vi "S4GUI_002.vi"(7 "Tab ObsEng":enum32{"Obs", "CCD modes", "Eng"}(tab)) -> ()   [LabVIEW 2018] (continued)
            n1697 = call "Write AcquisitionB.vi"("error in (no error)"=w3189, "Acquisition.lvclass"=w3190, "S4ACS_GUI in"=w3177) -> ("error out"=w3136:errorcluster, "S4ACS_GUI out"=w3135:refnum<class "S4GUI.lvclass">)  [unwired: 7 in]
            n1698 = call-dynamic "Read AcquisitionC.vi"("error in (no error)"=w3136, "S4ACS_GUI in"=w3135) -> ("error out"=w3173:errorcluster, "Acquisition.lvclass"=w3175:refnum<class "Acquisition.lvclass">, "S4ACS_GUI out"=w3176:refnum<class "S4GUI.lvclass">)  [unwired: 7 in]
            n1699 = call-dynamic "Read Channel.vi"("error in (no error)"=w3173, "Acquisition in"=w3175) -> ("error out"=w3160:errorcluster, "Channel.lvclass"=w3162:refnum<class "Channel.lvclass">, "Acquisition out"=w3174:refnum<class "Acquisition.lvclass">)  [unwired: 7 in]
            n1700 = call "Write section_name.vi"("error in (no error)"=w3160, "section_name"="CCD_ACS3", "Channel in"=w3162) -> ("error out"=w3159:errorcluster, "Channel out"=w3161:refnum<class "Channel.lvclass">)  [unwired: 7 in]
            n1701 = call-dynamic "load config.vi"("error in (no error)"=w3159, "cfg file name"=w3127, "Channel in"=w3161) -> ("error out"=w3117:errorcluster, "Channel out"=w3115:refnum<class "Channel.lvclass">)  [unwired: 7 in]
            n1702 = call-dynamic "save config.vi"("error in (no error)"=w3117, "file config"="lastsaved.cfg", "Channel in"=w3115) -> ("error out"=w3116:errorcluster, "Channel out"=w3114:refnum<class "Channel.lvclass">)  [unwired: 7 in]
            n1703 = call-dynamic "Read State Machine.vi"("error in (no error)"=w3116, "Device in"=w3114) -> ("error out"=w3169:errorcluster, "State Machine.lvclass"=w3171:refnum<class "State Machine.lvclass">, "Device out"=w3172:refnum<class "Channel.lvclass">)  [unwired: 7 in]
            n1704 = call-dynamic "Write State.vi"("error in (no error)"=w3169, "State"=60, "State Machine in"=w3171) -> ("error out"=w3168:errorcluster, "State Machine out"=w3170:refnum<class "State Machine.lvclass">)  [unwired: 7 in]
            n1705 = call-dynamic "Write State Machine.vi"("error in (no error)"=w3168, "State Machine.lvclass"=w3170, "Device in"=w3172) -> ("error out"=w3165:errorcluster, "Device out"=w3166:refnum<class "Channel.lvclass">)  [unwired: 7 in]
            n1706 = call-dynamic "Write Channel.vi"("error in (no error)"=w3165, "Channel.lvclass"=w3166, "Acquisition in"=w3174) -> ("error out"=w3164:errorcluster, "Acquisition out"=w3163:refnum<class "Acquisition.lvclass">)  [unwired: 7 in]
            n1707 = call-dynamic "Write AcquisitionC.vi"("error in (no error)"=w3164, "Acquisition.lvclass"=w3163, "S4ACS_GUI in"=w3176) -> ("error out"=w3134:errorcluster, "S4ACS_GUI out"=w3133:refnum<class "S4GUI.lvclass">)  [unwired: 7 in]
            n1708 = call-dynamic "Read AcquisitionD.vi"("error in (no error)"=w3134, "S4ACS_GUI in"=w3133) -> ("error out"=w3142:errorcluster, "Acquisition.lvclass"=w3140:refnum<class "Acquisition.lvclass">, "S4ACS_GUI out"=w3139:refnum<class "S4GUI.lvclass">)  [unwired: 7 in]
            n1709 = call-dynamic "Read Channel.vi"("error in (no error)"=w3142, "Acquisition in"=w3140) -> ("error out"=w3155:errorcluster, "Channel.lvclass"=w3153:refnum<class "Channel.lvclass">, "Acquisition out"=w3141:refnum<class "Acquisition.lvclass">)  [unwired: 7 in]
            n1710 = call "Write section_name.vi"("error in (no error)"=w3155, "section_name"="CCD_ACS4", "Channel in"=w3153) -> ("error out"=w3156:errorcluster, "Channel out"=w3154:refnum<class "Channel.lvclass">)  [unwired: 7 in]
            n1711 = call-dynamic "load config.vi"("error in (no error)"=w3156, "cfg file name"=w3127, "Channel in"=w3154) -> ("error out"=w3113:errorcluster, "Channel out"=w3111:refnum<class "Channel.lvclass">)  [unwired: 7 in]
            n1712 = call-dynamic "save config.vi"("error in (no error)"=w3113, "file config"="lastsaved.cfg", "Channel in"=w3111) -> ("error out"=w3112:errorcluster, "Channel out"=w3110:refnum<class "Channel.lvclass">)  [unwired: 7 in]
            n1713 = call-dynamic "Read State Machine.vi"("error in (no error)"=w3112, "Device in"=w3110) -> ("error out"=w3146:errorcluster, "State Machine.lvclass"=w3144:refnum<class "State Machine.lvclass">, "Device out"=w3143:refnum<class "Channel.lvclass">)  [unwired: 7 in]
            n1714 = call-dynamic "Write State.vi"("error in (no error)"=w3146, "State"=60, "State Machine in"=w3144) -> ("error out"=w3147:errorcluster, "State Machine out"=w3145:refnum<class "State Machine.lvclass">)  [unwired: 7 in]
            n1715 = call-dynamic "Write State Machine.vi"("error in (no error)"=w3147, "State Machine.lvclass"=w3145, "Device in"=w3143) -> ("error out"=w3150:errorcluster, "Device out"=w3149:refnum<class "Channel.lvclass">)  [unwired: 7 in]
            n1716 = call-dynamic "Write Channel.vi"("error in (no error)"=w3150, "Channel.lvclass"=w3149, "Acquisition in"=w3141) -> ("error out"=w3151:errorcluster, "Acquisition out"=w3152:refnum<class "Acquisition.lvclass">)  [unwired: 7 in]
            n1717 = call-dynamic "Write AcquisitionD.vi"("error in (no error)"=w3151, "Acquisition.lvclass"=w3152, "S4ACS_GUI in"=w3139) -> ("error out"=w3130:errorcluster, "S4ACS_GUI out"=w3132:refnum<class "S4GUI.lvclass">)  [unwired: 7 in]
            n1718 = Unbundle By Name(w3083) -> ("INITIAL_LINE"=w3104:u16, "INITIAL_COLUMN"=w3103:u16, "FINAL_LINE"=w3102:u16, "FINAL_COLUMN"=w3101:u16, "VBIN"=w3100:u16, "HBIN"=w3099:u16, "PREAMP"=w3098:u8, "EM_GAIN"=w3097:u16, "READOUT_RATE"=w3096:u8, "SHUTTER_OPENING_TIME"=w3095:u16, "SHUTTER_CLOSING_TIME"=w3094:u16, "VERTICAL_SHIFT_SPEED"=w3084:u8, "READ_MODE"=w3093:u8, "VERTICAL_CLOCK_VOLTAGE"=w3092:u8, "AD_CHANNEL"=w3091:u32, "SHUTTER_MODE"=w3090:u8, "SHUTTER_TTL"=w3089:u8, "TRIGGER_MODE"=w3088:u8, "FRAME_TRANSFER"=w3087:bool, "ACQUISITION_MODE"=w3086:u8, "EM_MODE"=w3085:u8)
            n1719 = call "Write cfg file.vi"("error in (no error)"=w3130, "cfg file"=w3127, "S4ACS_GUI in"=w3132) -> ("error out"=w3129:errorcluster, "S4ACS_GUI out"=w3131:refnum<class "S4GUI.lvclass">)  [unwired: 7 in]
            n1720 = local read "Input Cluster"() -> (w3106:T8)
            n1721 = Bundle By Name(cluster=w3106, "Parameters.Image \nInitial Line"=w3104, "Parameters.Image\nInitial Column"=w3103, "Parameters.Image\nFinal Line"=w3102, "Parameters.Image\nFInal Column"=w3101, "Parameters.Vertical\nBinning"=w3100, "Parameters.Horizontal\nBinning"=w3099, "Parameters.Pre-amplification\nGain"=w3098, "Parameters.CCD\nEM Gain"=w3097, "Parameters.Readout\nRate"=w3096, "Parameters.Shutter\nOpenning Time"=w3095, "Parameters.Shutter\nClosing Time"=w3094, "Parameters.Vertical\nShift Speed"=w3084, "Parameters.Read\nMode"=w3093, "Parameters.Vertical\nClock Voltage"=w3092, "Parameters.A/D \nChannel"=w3091, "Parameters.Shutter\nMode"=w3090, "Parameters.Shutter\nTTL"=w3089, "Parameters.Trigger\nMode"=w3088, "Parameters.Frame\nTransfer"=w3087, "Parameters.Acquisition\nMode"=w3086, "Parameters.CCD \nEM Mode"=w3085) -> (w3105:T8)
            n1722 = local write "Input Cluster"(w3105) -> ()
          }
          frame True {
          }
        }
      }
      event "Save As Button": Value Change {
        n1723 = event-data() -> ()  [unwired: 1 in, 6 out]
        n1724 = disable-structure shown="Enabled" {
          disable-tunnel: [w3231 w3243] -> w3220
          disable-tunnel: w3219 -> [w3230 _]
          disable-tunnel: [w3224 w3241] -> w3218
          frame Disabled {
            n1725 = String To Path(string="C:\\Users\\observer\\sparc4\\s4gui\\Config" ("default name")) -> (path=w3226:path)
            n1726 = call "File Dialog2"("start path"=w3226, "prompt"="Select file...", "button label"="Save", "default name"="lastsaved.cfg", "error in"=w3230, "pattern (all files)"="*.cfg") -> ("selected path"=w3225:path, "cancelled"=w3231:bool, "error out"=→"error out 3":errorcluster)  [unwired: 6 in, 1 out]
            n1727 = Strip Path(path=w3225) -> (name=w3224:string)  [unwired: 1 out]
          }
          frame Enabled {
            w3245 = ".cfg" ("regular expression")
            n1728 = Match Pattern(string="savefile", regular expression=w3245) -> (before substring=w3240:string, match substring=w3244:string)  [unwired: 1 in, 2 out]
            n1729 = String Length(string=w3240) -> (length=w3239:i32)
            n1730 = Equal?(x=w3244, y=w3245) -> (x = y?=w3235:bool)
            n1731 = Less?(x=w3239, y=20) -> (x < y?=w3236:bool)
            n1732 = And(x=w3236, y=w3235) -> (x .and. y?=w3237:bool)
            n1733 = case shown="False" w3237 {
              tunnel: w3240 -> [_ w3258]
              tunnel: w3244 -> [_ w3257]
              tunnel: [TRUE ("cancelled") FALSE ("cancelled")] -> w3243
              tunnel: [w3248 w3256] -> w3241
              tunnel: [w3248 w3256] -> w3242
              frame False {
                w3248 = "lastsaved.cfg" ("savefile")
                n1734 = One Button Dialog(message="Invalid file name!\nFile name length must be less than 20 characters\nand must contain .cfg ending." ("savefile")) -> ()  [unwired: 1 in, 1 out]
              }
              frame True {
                n1735 = call <vilib>:"Trim Whitespace.vi"("string"=w3258) -> ("trimmed string"=w3255:string)  [unwired: 1 in]
                n1736 = call <vilib>:"Space Constant.vi"() -> ("String"=w3253:string)
                n1737 = To Lower Case(string=w3255) -> (all lower case string=w3251:string)
                n1738 = Search and Replace String(replace all?=TRUE ("replace all? (F)"), input string=w3251, search string=w3253, replace string="" ("replace string (\"\")")) -> (result string=w3250:string)  [unwired: 4 in, 3 out]
                n1739 = Concatenate Strings(w3250, w3257) -> (w3256:string)
              }
            }
            n1740 = local write "savefile"(w3242) -> ()
          }
        }
        n1741 = case shown="False" w3220 {
          tunnel: w3223 -> [w3324 w3326]
          tunnel: [w3272 w3326] -> w3222
          tunnel: [w3270 w3325] -> w3221
          tunnel: w3219 -> [w3269 w3325]
          tunnel: w3218 -> [w3268 _]
          frame False {
            n1742 = call-dynamic "Read AcquisitionA.vi"("error in (no error)"=w3269, "S4ACS_GUI in"=w3324) -> ("error out"=w3320:errorcluster, "Acquisition.lvclass"=w3322:refnum<class "Acquisition.lvclass">, "S4ACS_GUI out"=w3323:refnum<class "S4GUI.lvclass">)  [unwired: 7 in]
            n1743 = call-dynamic "Read Channel.vi"("error in (no error)"=w3320, "Acquisition in"=w3322) -> ("error out"=w3315:errorcluster, "Channel.lvclass"=w3317:refnum<class "Channel.lvclass">, "Acquisition out"=w3321:refnum<class "Acquisition.lvclass">)  [unwired: 7 in]
            n1744 = call "Write section_name.vi"("error in (no error)"=w3315, "section_name"="CCD_ACS1", "Channel in"=w3317) -> ("error out"=w3314:errorcluster, "Channel out"=w3316:refnum<class "Channel.lvclass">)  [unwired: 7 in]
            n1745 = call-dynamic "save config.vi"("error in (no error)"=w3314, "file config"=w3268, "Channel in"=w3316) -> ("error out"=w3266:errorcluster, "Channel out"=w3267:refnum<class "Channel.lvclass">)  [unwired: 7 in]
            n1746 = call-dynamic "Write Channel.vi"("error in (no error)"=w3266, "Channel.lvclass"=w3267, "Acquisition in"=w3321) -> ("error out"=w3319:errorcluster, "Acquisition out"=w3318:refnum<class "Acquisition.lvclass">)  [unwired: 7 in]
            n1747 = call-dynamic "Write AcquisitionA.vi"("error in (no error)"=w3319, "Acquisition.lvclass"=w3318, "S4ACS_GUI in"=w3323) -> ("error out"=w3279:errorcluster, "S4ACS_GUI out"=w3278:refnum<class "S4GUI.lvclass">)  [unwired: 7 in]
            n1748 = call "Read AcquisitionB.vi"("error in (no error)"=w3279, "S4ACS_GUI in"=w3278) -> ("error out"=w3305:errorcluster, "Acquisition.lvclass"=w3303:refnum<class "Acquisition.lvclass">, "S4ACS_GUI out"=w3302:refnum<class "S4GUI.lvclass">)  [unwired: 7 in]
            n1749 = call-dynamic "Read Channel.vi"("error in (no error)"=w3305, "Acquisition in"=w3303) -> ("error out"=w3310:errorcluster, "Channel.lvclass"=w3308:refnum<class "Channel.lvclass">, "Acquisition out"=w3304:refnum<class "Acquisition.lvclass">)  [unwired: 7 in]
            n1750 = call "Write section_name.vi"("error in (no error)"=w3310, "section_name"="CCD_ACS2", "Channel in"=w3308) -> ("error out"=w3311:errorcluster, "Channel out"=w3309:refnum<class "Channel.lvclass">)  [unwired: 7 in]
            n1751 = call-dynamic "save config.vi"("error in (no error)"=w3311, "file config"=w3268, "Channel in"=w3309) -> ("error out"=w3260:errorcluster, "Channel out"=w3261:refnum<class "Channel.lvclass">)  [unwired: 7 in]
            n1752 = call-dynamic "Write Channel.vi"("error in (no error)"=w3260, "Channel.lvclass"=w3261, "Acquisition in"=w3304) -> ("error out"=w3306:errorcluster, "Acquisition out"=w3307:refnum<class "Acquisition.lvclass">)  [unwired: 7 in]
            n1753 = call "Write AcquisitionB.vi"("error in (no error)"=w3306, "Acquisition.lvclass"=w3307, "S4ACS_GUI in"=w3302) -> ("error out"=w3277:errorcluster, "S4ACS_GUI out"=w3276:refnum<class "S4GUI.lvclass">)  [unwired: 7 in]
            n1754 = call-dynamic "Read AcquisitionC.vi"("error in (no error)"=w3277, "S4ACS_GUI in"=w3276) -> ("error out"=w3298:errorcluster, "Acquisition.lvclass"=w3300:refnum<class "Acquisition.lvclass">, "S4ACS_GUI out"=w3301:refnum<class "S4GUI.lvclass">)  [unwired: 7 in]
            n1755 = call-dynamic "Read Channel.vi"("error in (no error)"=w3298, "Acquisition in"=w3300) -> ("error out"=w3293:errorcluster, "Channel.lvclass"=w3295:refnum<class "Channel.lvclass">, "Acquisition out"=w3299:refnum<class "Acquisition.lvclass">)  [unwired: 7 in]
            n1756 = call "Write section_name.vi"("error in (no error)"=w3293, "section_name"="CCD_ACS3", "Channel in"=w3295) -> ("error out"=w3292:errorcluster, "Channel out"=w3294:refnum<class "Channel.lvclass">)  [unwired: 7 in]
            n1757 = call-dynamic "save config.vi"("error in (no error)"=w3292, "file config"=w3268, "Channel in"=w3294) -> ("error out"=w3262:errorcluster, "Channel out"=w3263:refnum<class "Channel.lvclass">)  [unwired: 7 in]
            n1758 = call-dynamic "Write Channel.vi"("error in (no error)"=w3262, "Channel.lvclass"=w3263, "Acquisition in"=w3299) -> ("error out"=w3297:errorcluster, "Acquisition out"=w3296:refnum<class "Acquisition.lvclass">)  [unwired: 7 in]
            n1759 = call-dynamic "Write AcquisitionC.vi"("error in (no error)"=w3297, "Acquisition.lvclass"=w3296, "S4ACS_GUI in"=w3301) -> ("error out"=w3275:errorcluster, "S4ACS_GUI out"=w3274:refnum<class "S4GUI.lvclass">)  [unwired: 7 in]
            n1760 = call-dynamic "Read AcquisitionD.vi"("error in (no error)"=w3275, "S4ACS_GUI in"=w3274) -> ("error out"=w3283:errorcluster, "Acquisition.lvclass"=w3281:refnum<class "Acquisition.lvclass">, "S4ACS_GUI out"=w3280:refnum<class "S4GUI.lvclass">)  [unwired: 7 in]
            n1761 = call-dynamic "Read Channel.vi"("error in (no error)"=w3283, "Acquisition in"=w3281) -> ("error out"=w3288:errorcluster, "Channel.lvclass"=w3286:refnum<class "Channel.lvclass">, "Acquisition out"=w3282:refnum<class "Acquisition.lvclass">)  [unwired: 7 in]
            n1762 = call "Write section_name.vi"("error in (no error)"=w3288, "section_name"="CCD_ACS4", "Channel in"=w3286) -> ("error out"=w3289:errorcluster, "Channel out"=w3287:refnum<class "Channel.lvclass">)  [unwired: 7 in]
            n1763 = call-dynamic "save config.vi"("error in (no error)"=w3289, "file config"=w3268, "Channel in"=w3287) -> ("error out"=w3264:errorcluster, "Channel out"=w3265:refnum<class "Channel.lvclass">)  [unwired: 7 in]
            n1764 = call-dynamic "Write Channel.vi"("error in (no error)"=w3264, "Channel.lvclass"=w3265, "Acquisition in"=w3282) -> ("error out"=w3284:errorcluster, "Acquisition out"=w3285:refnum<class "Acquisition.lvclass">)  [unwired: 7 in]
            n1765 = call-dynamic "Write AcquisitionD.vi"("error in (no error)"=w3284, "Acquisition.lvclass"=w3285, "S4ACS_GUI in"=w3280) -> ("error out"=w3271:errorcluster, "S4ACS_GUI out"=w3273:refnum<class "S4GUI.lvclass">)  [unwired: 7 in]
            n1766 = call "Write cfg file.vi"("error in (no error)"=w3271, "cfg file"=w3268, "S4ACS_GUI in"=w3273) -> ("error out"=w3270:errorcluster, "S4ACS_GUI out"=w3272:refnum<class "S4GUI.lvclass">)  [unwired: 7 in]
          }
          frame True {
          }
        }
      }
      event "Load Default Button": Value Change {
        w3371 = "default.cfg" ("cfg file name")
        n1767 = event-data() -> ()  [unwired: 1 in, 6 out]
        n1768 = call-dynamic "Read AcquisitionA.vi"("error in (no error)"=w3461, "S4ACS_GUI in"=w3462) -> ("error out"=w3457:errorcluster, "Acquisition.lvclass"=w3459:refnum<class "Acquisition.lvclass">, "S4ACS_GUI out"=w3460:refnum<class "S4GUI.lvclass">)  [unwired: 7 in]
        n1769 = call-dynamic "Read Channel.vi"("error in (no error)"=w3457, "Acquisition in"=w3459) -> ("error out"=w3444:errorcluster, "Channel.lvclass"=w3446:refnum<class "Channel.lvclass">, "Acquisition out"=w3458:refnum<class "Acquisition.lvclass">)  [unwired: 7 in]
        n1770 = call "Write section_name.vi"("error in (no error)"=w3444, "section_name"="CCD_ACS1", "Channel in"=w3446) -> ("error out"=w3443:errorcluster, "Channel out"=w3445:refnum<class "Channel.lvclass">)  [unwired: 7 in]
        n1771 = call-dynamic "load config.vi"("error in (no error)"=w3443, "cfg file name"=w3371, "Channel in"=w3445) -> ("error out"=w3369:errorcluster, "Channel out"=w3370:refnum<class "Channel.lvclass">)  [unwired: 7 in]
        n1772 = call-dynamic "save config.vi"("error in (no error)"=w3369, "file config"="lastsaved.cfg", "Channel in"=w3370) -> ("error out"=w3328:errorcluster, "Channel out"=w3329:refnum<class "Channel.lvclass">)  [unwired: 7 in]
        n1773 = call-dynamic "Read target cluster.vi"("error in (no error)"=w3328, "Channel in"=w3329) -> ("target cluster"=w3327:T31)  [unwired: 7 in, 2 out]
        n1774 = call-dynamic "Read State Machine.vi"("error in (no error)"=w3328, "Device in"=w3329) -> ("error out"=w3453:errorcluster, "State Machine.lvclass"=w3455:refnum<class "State Machine.lvclass">, "Device out"=w3456:refnum<class "Channel.lvclass">)  [unwired: 7 in]
        n1775 = call-dynamic "Write State.vi"("error in (no error)"=w3453, "State"=60, "State Machine in"=w3455) -> ("error out"=w3452:errorcluster, "State Machine out"=w3454:refnum<class "State Machine.lvclass">)  [unwired: 7 in]
        n1776 = call-dynamic "Write State Machine.vi"("error in (no error)"=w3452, "State Machine.lvclass"=w3454, "Device in"=w3456) -> ("error out"=w3449:errorcluster, "Device out"=w3450:refnum<class "Channel.lvclass">)  [unwired: 7 in]
        n1777 = call-dynamic "Write Channel.vi"("error in (no error)"=w3449, "Channel.lvclass"=w3450, "Acquisition in"=w3458) -> ("error out"=w3448:errorcluster, "Acquisition out"=w3447:refnum<class "Acquisition.lvclass">)  [unwired: 7 in]
        n1778 = call-dynamic "Write AcquisitionA.vi"("error in (no error)"=w3448, "Acquisition.lvclass"=w3447, "S4ACS_GUI in"=w3460) -> ("error out"=w3381:errorcluster, "S4ACS_GUI out"=w3380:refnum<class "S4GUI.lvclass">)  [unwired: 7 in]
        n1779 = call "Read AcquisitionB.vi"("error in (no error)"=w3381, "S4ACS_GUI in"=w3380) -> ("error out"=w3425:errorcluster, "Acquisition.lvclass"=w3423:refnum<class "Acquisition.lvclass">, "S4ACS_GUI out"=w3422:refnum<class "S4GUI.lvclass">)  [unwired: 7 in]
        n1780 = call-dynamic "Read Channel.vi"("error in (no error)"=w3425, "Acquisition in"=w3423) -> ("error out"=w3439:errorcluster, "Channel.lvclass"=w3437:refnum<class "Channel.lvclass">, "Acquisition out"=w3424:refnum<class "Acquisition.lvclass">)  [unwired: 7 in]
        n1781 = call "Write section_name.vi"("error in (no error)"=w3439, "section_name"="CCD_ACS2", "Channel in"=w3437) -> ("error out"=w3440:errorcluster, "Channel out"=w3438:refnum<class "Channel.lvclass">)  [unwired: 7 in]
        n1782 = call-dynamic "load config.vi"("error in (no error)"=w3440, "cfg file name"="default.cfg", "Channel in"=w3438) -> ("error out"=w3366:errorcluster, "Channel out"=w3364:refnum<class "Channel.lvclass">)  [unwired: 7 in]
        n1783 = call-dynamic "save config.vi"("error in (no error)"=w3366, "file config"="lastsaved.cfg", "Channel in"=w3364) -> ("error out"=w3365:errorcluster, "Channel out"=w3363:refnum<class "Channel.lvclass">)  [unwired: 7 in]
        n1784 = call-dynamic "Read State Machine.vi"("error in (no error)"=w3365, "Device in"=w3363) -> ("error out"=w3429:errorcluster, "State Machine.lvclass"=w3427:refnum<class "State Machine.lvclass">, "Device out"=w3426:refnum<class "Channel.lvclass">)  [unwired: 7 in]
        n1785 = call-dynamic "Write State.vi"("error in (no error)"=w3429, "State"=60, "State Machine in"=w3427) -> ("error out"=w3430:errorcluster, "State Machine out"=w3428:refnum<class "State Machine.lvclass">)  [unwired: 7 in]
        n1786 = call-dynamic "Write State Machine.vi"("error in (no error)"=w3430, "State Machine.lvclass"=w3428, "Device in"=w3426) -> ("error out"=w3433:errorcluster, "Device out"=w3432:refnum<class "Channel.lvclass">)  [unwired: 7 in]
        n1787 = call-dynamic "Write Channel.vi"("error in (no error)"=w3433, "Channel.lvclass"=w3432, "Acquisition in"=w3424) -> ("error out"=w3434:errorcluster, "Acquisition out"=w3435:refnum<class "Acquisition.lvclass">)  [unwired: 7 in]
        n1788 = call "Write AcquisitionB.vi"("error in (no error)"=w3434, "Acquisition.lvclass"=w3435, "S4ACS_GUI in"=w3422) -> ("error out"=w3379:errorcluster, "S4ACS_GUI out"=w3378:refnum<class "S4GUI.lvclass">)  [unwired: 7 in]
        n1789 = call-dynamic "Read AcquisitionC.vi"("error in (no error)"=w3379, "S4ACS_GUI in"=w3378) -> ("error out"=w3418:errorcluster, "Acquisition.lvclass"=w3420:refnum<class "Acquisition.lvclass">, "S4ACS_GUI out"=w3421:refnum<class "S4GUI.lvclass">)  [unwired: 7 in]
        n1790 = call-dynamic "Read Channel.vi"("error in (no error)"=w3418, "Acquisition in"=w3420) -> ("error out"=w3404:errorcluster, "Channel.lvclass"=w3406:refnum<class "Channel.lvclass">, "Acquisition out"=w3419:refnum<class "Acquisition.lvclass">)  [unwired: 7 in]
        n1791 = call "Write section_name.vi"("error in (no error)"=w3404, "section_name"="CCD_ACS3", "Channel in"=w3406) -> ("error out"=w3403:errorcluster, "Channel out"=w3405:refnum<class "Channel.lvclass">)  [unwired: 7 in]
        n1792 = call-dynamic "load config.vi"("error in (no error)"=w3403, "cfg file name"="default.cfg", "Channel in"=w3405) -> ("error out"=w3360:errorcluster, "Channel out"=w3361:refnum<class "Channel.lvclass">)  [unwired: 7 in]
        n1793 = call-dynamic "save config.vi"("error in (no error)"=w3360, "file config"="lastsaved.cfg", "Channel in"=w3361) -> ("error out"=w3358:errorcluster, "Channel out"=w3359:refnum<class "Channel.lvclass">)  [unwired: 7 in]
        n1794 = call-dynamic "Read State Machine.vi"("error in (no error)"=w3358, "Device in"=w3359) -> ("error out"=w3414:errorcluster, "State Machine.lvclass"=w3416:refnum<class "State Machine.lvclass">, "Device out"=w3417:refnum<class "Channel.lvclass">)  [unwired: 7 in]
        n1795 = call-dynamic "Write State.vi"("error in (no error)"=w3414, "State"=60, "State Machine in"=w3416) -> ("error out"=w3413:errorcluster, "State Machine out"=w3415:refnum<class "State Machine.lvclass">)  [unwired: 7 in]
        n1796 = call-dynamic "Write State Machine.vi"("error in (no error)"=w3413, "State Machine.lvclass"=w3415, "Device in"=w3417) -> ("error out"=w3410:errorcluster, "Device out"=w3411:refnum<class "Channel.lvclass">)  [unwired: 7 in]
        n1797 = call-dynamic "Write Channel.vi"("error in (no error)"=w3410, "Channel.lvclass"=w3411, "Acquisition in"=w3419) -> ("error out"=w3409:errorcluster, "Acquisition out"=w3408:refnum<class "Acquisition.lvclass">)  [unwired: 7 in]
        n1798 = call-dynamic "Write AcquisitionC.vi"("error in (no error)"=w3409, "Acquisition.lvclass"=w3408, "S4ACS_GUI in"=w3421) -> ("error out"=w3377:errorcluster, "S4ACS_GUI out"=w3376:refnum<class "S4GUI.lvclass">)  [unwired: 7 in]
        n1799 = call-dynamic "Read AcquisitionD.vi"("error in (no error)"=w3377, "S4ACS_GUI in"=w3376) -> ("error out"=w3385:errorcluster, "Acquisition.lvclass"=w3383:refnum<class "Acquisition.lvclass">, "S4ACS_GUI out"=w3382:refnum<class "S4GUI.lvclass">)  [unwired: 7 in]
        n1800 = call-dynamic "Read Channel.vi"("error in (no error)"=w3385, "Acquisition in"=w3383) -> ("error out"=w3399:errorcluster, "Channel.lvclass"=w3397:refnum<class "Channel.lvclass">, "Acquisition out"=w3384:refnum<class "Acquisition.lvclass">)  [unwired: 7 in]
        n1801 = call "Write section_name.vi"("error in (no error)"=w3399, "section_name"="CCD_ACS4", "Channel in"=w3397) -> ("error out"=w3400:errorcluster, "Channel out"=w3398:refnum<class "Channel.lvclass">)  [unwired: 7 in]
        n1802 = call-dynamic "load config.vi"("error in (no error)"=w3400, "cfg file name"="default.cfg", "Channel in"=w3398) -> ("error out"=w3356:errorcluster, "Channel out"=w3355:refnum<class "Channel.lvclass">)  [unwired: 7 in]
        n1803 = call-dynamic "save config.vi"("error in (no error)"=w3356, "file config"="lastsaved.cfg", "Channel in"=w3355) -> ("error out"=w3353:errorcluster, "Channel out"=w3354:refnum<class "Channel.lvclass">)  [unwired: 7 in]
        n1804 = call-dynamic "Read State Machine.vi"("error in (no error)"=w3353, "Device in"=w3354) -> ("error out"=w3389:errorcluster, "State Machine.lvclass"=w3387:refnum<class "State Machine.lvclass">, "Device out"=w3386:refnum<class "Channel.lvclass">)  [unwired: 7 in]
        n1805 = call-dynamic "Write State.vi"("error in (no error)"=w3389, "State"=60, "State Machine in"=w3387) -> ("error out"=w3390:errorcluster, "State Machine out"=w3388:refnum<class "State Machine.lvclass">)  [unwired: 7 in]
        n1806 = call-dynamic "Write State Machine.vi"("error in (no error)"=w3390, "State Machine.lvclass"=w3388, "Device in"=w3386) -> ("error out"=w3393:errorcluster, "Device out"=w3392:refnum<class "Channel.lvclass">)  [unwired: 7 in]
        n1807 = call-dynamic "Write Channel.vi"("error in (no error)"=w3393, "Channel.lvclass"=w3392, "Acquisition in"=w3384) -> ("error out"=w3394:errorcluster, "Acquisition out"=w3395:refnum<class "Acquisition.lvclass">)  [unwired: 7 in]
        n1808 = call-dynamic "Write AcquisitionD.vi"("error in (no error)"=w3394, "Acquisition.lvclass"=w3395, "S4ACS_GUI in"=w3382) -> ("error out"=w3373:errorcluster, "S4ACS_GUI out"=w3375:refnum<class "S4GUI.lvclass">)  [unwired: 7 in]
        n1809 = Unbundle By Name(w3327) -> ("INITIAL_LINE"=w3332:u16, "INITIAL_COLUMN"=w3333:u16, "FINAL_LINE"=w3334:u16, "FINAL_COLUMN"=w3335:u16, "VBIN"=w3336:u16, "HBIN"=w3337:u16, "PREAMP"=w3338:u8, "EM_GAIN"=w3339:u16, "READOUT_RATE"=w3340:u8, "SHUTTER_OPENING_TIME"=w3341:u16, "SHUTTER_CLOSING_TIME"=w3342:u16, "VERTICAL_SHIFT_SPEED"=w3352:u8, "READ_MODE"=w3343:u8, "VERTICAL_CLOCK_VOLTAGE"=w3344:u8, "AD_CHANNEL"=w3345:u32, "SHUTTER_MODE"=w3346:u8, "SHUTTER_TTL"=w3347:u8, "TRIGGER_MODE"=w3348:u8, "FRAME_TRANSFER"=w3349:bool, "ACQUISITION_MODE"=w3350:u8, "EM_MODE"=w3351:u8)
        n1810 = call "Write cfg file.vi"("error in (no error)"=w3373, "cfg file"=w3371, "S4ACS_GUI in"=w3375) -> ("error out"=w3372:errorcluster, "S4ACS_GUI out"=w3374:refnum<class "S4GUI.lvclass">)  [unwired: 7 in]
        n1811 = local read "Input Cluster"() -> (w3330:T8)
        n1812 = Bundle By Name(cluster=w3330, "Parameters.Image \nInitial Line"=w3332, "Parameters.Image\nInitial Column"=w3333, "Parameters.Image\nFinal Line"=w3334, "Parameters.Image\nFInal Column"=w3335, "Parameters.Vertical\nBinning"=w3336, "Parameters.Horizontal\nBinning"=w3337, "Parameters.Pre-amplification\nGain"=w3338, "Parameters.CCD\nEM Gain"=w3339, "Parameters.Readout\nRate"=w3340, "Parameters.Shutter\nOpenning Time"=w3341, "Parameters.Shutter\nClosing Time"=w3342, "Parameters.Vertical\nShift Speed"=w3352, "Parameters.Read\nMode"=w3343, "Parameters.Vertical\nClock Voltage"=w3344, "Parameters.A/D \nChannel"=w3345, "Parameters.Shutter\nMode"=w3346, "Parameters.Shutter\nTTL"=w3347, "Parameters.Trigger\nMode"=w3348, "Parameters.Frame\nTransfer"=w3349, "Parameters.Acquisition\nMode"=w3350, "Parameters.CCD \nEM Mode"=w3351) -> (w3331:T8)
        n1813 = local write "Input Cluster"(w3331) -> ()
      }
      event "Restore Default ch2": Value Change {
        n1814 = event-data() -> ()  [unwired: 1 in, 6 out]
        n1815 = call "Read AcquisitionB.vi"("error in (no error)"=w3493, "S4ACS_GUI in"=w3494) -> ("error out"=w3489:errorcluster, "Acquisition.lvclass"=w3491:refnum<class "Acquisition.lvclass">, "S4ACS_GUI out"=w3492:refnum<class "S4GUI.lvclass">)  [unwired: 7 in]
        n1816 = call-dynamic "Read Channel.vi"("error in (no error)"=w3489, "Acquisition in"=w3491) -> ("error out"=w3476:errorcluster, "Channel.lvclass"=w3478:refnum<class "Channel.lvclass">, "Acquisition out"=w3490:refnum<class "Acquisition.lvclass">)  [unwired: 7 in]
        n1817 = call "Write section_name.vi"("error in (no error)"=w3476, "section_name"="CCD_ACS2", "Channel in"=w3478) -> ("error out"=w3475:errorcluster, "Channel out"=w3477:refnum<class "Channel.lvclass">)  [unwired: 7 in]
        n1818 = call-dynamic "load config.vi"("error in (no error)"=w3475, "cfg file name"="default.cfg", "Channel in"=w3477) -> ("error out"=w3473:errorcluster, "Channel out"=w3474:refnum<class "Channel.lvclass">)  [unwired: 7 in]
        n1819 = call-dynamic "Read State Machine.vi"("error in (no error)"=w3473, "Device in"=w3474) -> ("error out"=w3485:errorcluster, "State Machine.lvclass"=w3487:refnum<class "State Machine.lvclass">, "Device out"=w3488:refnum<class "Channel.lvclass">)  [unwired: 7 in]
        n1820 = call-dynamic "Write State.vi"("error in (no error)"=w3485, "State"=60, "State Machine in"=w3487) -> ("error out"=w3484:errorcluster, "State Machine out"=w3486:refnum<class "State Machine.lvclass">)  [unwired: 7 in]
        n1821 = call-dynamic "Write State Machine.vi"("error in (no error)"=w3484, "State Machine.lvclass"=w3486, "Device in"=w3488) -> ("error out"=w3469:errorcluster, "Device out"=w3466:refnum<class "Channel.lvclass">)  [unwired: 7 in]
        n1822 = call "Write section_name.vi"("error in (no error)"=w3469, "section_name"="CCD_ACS2", "Channel in"=w3466) -> ("error out"=w3470:errorcluster, "Channel out"=w3465:refnum<class "Channel.lvclass">)  [unwired: 7 in]
        n1823 = call-dynamic "save config.vi"("error in (no error)"=w3470, "file config"="lastsaved.cfg", "Channel in"=w3465) -> ("error out"=w3468:errorcluster, "Channel out"=w3464:refnum<class "Channel.lvclass">)  [unwired: 7 in]
        n1824 = call-dynamic "Write Channel.vi"("error in (no error)"=w3468, "Channel.lvclass"=w3464, "Acquisition in"=w3490) -> ("error out"=w3482:errorcluster, "Acquisition out"=w3481:refnum<class "Acquisition.lvclass">)  [unwired: 7 in]
        n1825 = call "Write AcquisitionB.vi"("error in (no error)"=w3482, "Acquisition.lvclass"=w3481, "S4ACS_GUI in"=w3492) -> ("error out"=w3480:errorcluster, "S4ACS_GUI out"=w3471:refnum<class "S4GUI.lvclass">)  [unwired: 7 in]
      }
      event "Restore Default ch3": Value Change {
        n1826 = event-data() -> ()  [unwired: 1 in, 6 out]
        n1827 = call-dynamic "Read AcquisitionC.vi"("error in (no error)"=w3525, "S4ACS_GUI in"=w3526) -> ("error out"=w3521:errorcluster, "Acquisition.lvclass"=w3523:refnum<class "Acquisition.lvclass">, "S4ACS_GUI out"=w3524:refnum<class "S4GUI.lvclass">)  [unwired: 7 in]
        n1828 = call-dynamic "Read Channel.vi"("error in (no error)"=w3521, "Acquisition in"=w3523) -> ("error out"=w3508:errorcluster, "Channel.lvclass"=w3510:refnum<class "Channel.lvclass">, "Acquisition out"=w3522:refnum<class "Acquisition.lvclass">)  [unwired: 7 in]
        n1829 = call "Write section_name.vi"("error in (no error)"=w3508, "section_name"="CCD_ACS3", "Channel in"=w3510) -> ("error out"=w3507:errorcluster, "Channel out"=w3509:refnum<class "Channel.lvclass">)  [unwired: 7 in]
        n1830 = call-dynamic "load config.vi"("error in (no error)"=w3507, "cfg file name"="default.cfg", "Channel in"=w3509) -> ("error out"=w3505:errorcluster, "Channel out"=w3506:refnum<class "Channel.lvclass">)  [unwired: 7 in]
        n1831 = call-dynamic "Read State Machine.vi"("error in (no error)"=w3505, "Device in"=w3506) -> ("error out"=w3517:errorcluster, "State Machine.lvclass"=w3519:refnum<class "State Machine.lvclass">, "Device out"=w3520:refnum<class "Channel.lvclass">)  [unwired: 7 in]
        n1832 = call-dynamic "Write State.vi"("error in (no error)"=w3517, "State"=60, "State Machine in"=w3519) -> ("error out"=w3516:errorcluster, "State Machine out"=w3518:refnum<class "State Machine.lvclass">)  [unwired: 7 in]
        n1833 = call-dynamic "Write State Machine.vi"("error in (no error)"=w3516, "State Machine.lvclass"=w3518, "Device in"=w3520) -> ("error out"=w3496:errorcluster, "Device out"=w3498:refnum<class "Channel.lvclass">)  [unwired: 7 in]
        n1834 = call "Write section_name.vi"("error in (no error)"=w3496, "section_name"="CCD_ACS3", "Channel in"=w3498) -> ("error out"=w3502:errorcluster, "Channel out"=w3497:refnum<class "Channel.lvclass">)  [unwired: 7 in]
        n1835 = call-dynamic "save config.vi"("error in (no error)"=w3502, "file config"="lastsaved.cfg", "Channel in"=w3497) -> ("error out"=w3495:errorcluster, "Channel out"=w3499:refnum<class "Channel.lvclass">)  [unwired: 7 in]
        n1836 = call-dynamic "Write Channel.vi"("error in (no error)"=w3495, "Channel.lvclass"=w3499, "Acquisition in"=w3522) -> ("error out"=w3514:errorcluster, "Acquisition out"=w3513:refnum<class "Acquisition.lvclass">)  [unwired: 7 in]
        n1837 = call-dynamic "Write AcquisitionC.vi"("error in (no error)"=w3514, "Acquisition.lvclass"=w3513, "S4ACS_GUI in"=w3524) -> ("error out"=w3512:errorcluster, "S4ACS_GUI out"=w3503:refnum<class "S4GUI.lvclass">)  [unwired: 7 in]
      }
      event "Restore Default ch4": Value Change {
        n1838 = event-data() -> ()  [unwired: 1 in, 6 out]
        n1839 = call-dynamic "Read AcquisitionD.vi"("error in (no error)"=w3557, "S4ACS_GUI in"=w3558) -> ("error out"=w3553:errorcluster, "Acquisition.lvclass"=w3555:refnum<class "Acquisition.lvclass">, "S4ACS_GUI out"=w3556:refnum<class "S4GUI.lvclass">)  [unwired: 7 in]
        n1840 = call-dynamic "Read Channel.vi"("error in (no error)"=w3553, "Acquisition in"=w3555) -> ("error out"=w3540:errorcluster, "Channel.lvclass"=w3542:refnum<class "Channel.lvclass">, "Acquisition out"=w3554:refnum<class "Acquisition.lvclass">)  [unwired: 7 in]
        n1841 = call "Write section_name.vi"("error in (no error)"=w3540, "section_name"="CCD_ACS4", "Channel in"=w3542) -> ("error out"=w3539:errorcluster, "Channel out"=w3541:refnum<class "Channel.lvclass">)  [unwired: 7 in]
        n1842 = call-dynamic "load config.vi"("error in (no error)"=w3539, "cfg file name"="default.cfg", "Channel in"=w3541) -> ("error out"=w3537:errorcluster, "Channel out"=w3538:refnum<class "Channel.lvclass">)  [unwired: 7 in]
        n1843 = call-dynamic "Read State Machine.vi"("error in (no error)"=w3537, "Device in"=w3538) -> ("error out"=w3549:errorcluster, "State Machine.lvclass"=w3551:refnum<class "State Machine.lvclass">, "Device out"=w3552:refnum<class "Channel.lvclass">)  [unwired: 7 in]
        n1844 = call-dynamic "Write State.vi"("error in (no error)"=w3549, "State"=60, "State Machine in"=w3551) -> ("error out"=w3548:errorcluster, "State Machine out"=w3550:refnum<class "State Machine.lvclass">)  [unwired: 7 in]
        n1845 = call-dynamic "Write State Machine.vi"("error in (no error)"=w3548, "State Machine.lvclass"=w3550, "Device in"=w3552) -> ("error out"=w3528:errorcluster, "Device out"=w3531:refnum<class "Channel.lvclass">)  [unwired: 7 in]
        n1846 = call "Write section_name.vi"("error in (no error)"=w3528, "section_name"="CCD_ACS4", "Channel in"=w3531) -> ("error out"=w3534:errorcluster, "Channel out"=w3530:refnum<class "Channel.lvclass">)  [unwired: 7 in]
        n1847 = call-dynamic "save config.vi"("error in (no error)"=w3534, "file config"="lastsaved.cfg", "Channel in"=w3530) -> ("error out"=w3527:errorcluster, "Channel out"=w3529:refnum<class "Channel.lvclass">)  [unwired: 7 in]
        n1848 = call-dynamic "Write Channel.vi"("error in (no error)"=w3527, "Channel.lvclass"=w3529, "Acquisition in"=w3554) -> ("error out"=w3546:errorcluster, "Acquisition out"=w3545:refnum<class "Acquisition.lvclass">)  [unwired: 7 in]
        n1849 = call-dynamic "Write AcquisitionD.vi"("error in (no error)"=w3546, "Acquisition.lvclass"=w3545, "S4ACS_GUI in"=w3556) -> ("error out"=w3544:errorcluster, "S4ACS_GUI out"=w3535:refnum<class "S4GUI.lvclass">)  [unwired: 7 in]
      }
      event "Copy to Input ch1": Value Change {
        w3559 = T12."Enabled" ("Disabled")
        n1850 = event-data() -> ()  [unwired: 1 in, 6 out]
        n1851 = call-dynamic "Read AcquisitionA.vi"("error in (no error)"=w3592, "S4ACS_GUI in"=w3593) -> ("error out"=w3588:errorcluster, "Acquisition.lvclass"=w3591:refnum<class "Acquisition.lvclass">, "S4ACS_GUI out"=w3560:refnum<class "S4GUI.lvclass">)  [unwired: 7 in]
        n1852 = call-dynamic "Read Channel.vi"("error in (no error)"=w3588, "Acquisition in"=w3591) -> ("error out"=w3587:errorcluster, "Channel.lvclass"=w3590:refnum<class "Channel.lvclass">)  [unwired: 7 in, 1 out]
        n1853 = call-dynamic "Read Interface.vi"("error in (no error)"=w3587, "Channel in"=w3590) -> ("error out"=w3586:errorcluster, "Interface.lvclass"=w3589:refnum<class "Interface.lvclass">)  [unwired: 7 in, 1 out]
        n1854 = call-dynamic "Get CCD_Config.vi"("error in (no error)"=w3586, "Interface in"=w3589) -> ("error out"=w3583:errorcluster, "output cluster"=w3582:T31)  [unwired: 7 in, 1 out]
        n1855 = Unbundle By Name(w3582) -> ("INITIAL_LINE"=w3581:u16, "INITIAL_COLUMN"=w3580:u16, "FINAL_LINE"=w3579:u16, "FINAL_COLUMN"=w3578:u16, "VBIN"=w3577:u16, "HBIN"=w3576:u16, "PREAMP"=w3575:u8, "EM_GAIN"=w3574:u16, "READOUT_RATE"=w3573:u8, "SHUTTER_OPENING_TIME"=w3572:u16, "SHUTTER_CLOSING_TIME"=w3571:u16, "VERTICAL_SHIFT_SPEED"=w3570:u8, "READ_MODE"=w3569:u8, "VERTICAL_CLOCK_VOLTAGE"=w3568:u8, "AD_CHANNEL"=w3567:u32, "SHUTTER_MODE"=w3566:u8, "SHUTTER_TTL"=w3565:u8, "TRIGGER_MODE"=w3564:u8, "FRAME_TRANSFER"=w3563:bool, "ACQUISITION_MODE"=w3562:u8, "EM_MODE"=w3561:u8)
        n1856 = local read "Input Cluster"() -> (w3585:T8)
        n1857 = Bundle By Name(cluster=w3585, "Parameters.Image \nInitial Line"=w3581, "Parameters.Image\nInitial Column"=w3580, "Parameters.Image\nFinal Line"=w3579, "Parameters.Image\nFInal Column"=w3578, "Parameters.Vertical\nBinning"=w3577, "Parameters.Horizontal\nBinning"=w3576, "Parameters.Pre-amplification\nGain"=w3575, "Parameters.CCD\nEM Gain"=w3574, "Parameters.Readout\nRate"=w3573, "Parameters.Shutter\nOpenning Time"=w3572, "Parameters.Shutter\nClosing Time"=w3571, "Parameters.Vertical\nShift Speed"=w3570, "Parameters.Read\nMode"=w3569, "Parameters.Vertical\nClock Voltage"=w3568, "Parameters.A/D \nChannel"=w3567, "Parameters.Shutter\nMode"=w3566, "Parameters.Shutter\nTTL"=w3565, "Parameters.Trigger\nMode"=w3564, "Parameters.Frame\nTransfer"=w3563, "Parameters.Acquisition\nMode"=w3562, "Parameters.CCD \nEM Mode"=w3561) -> (w3584:T8)
        n1858 = local write "Input Cluster"(w3584) -> ()
        n1859 = property on="Set from Input ch1" class="Bool"("DisabledEnum"=w3559) -> ()  [unwired: 2 in, 2 out]
        n1860 = property on="Set from Input ch3" class="Bool"("DisabledEnum"=w3559) -> ()  [unwired: 2 in, 2 out]
        n1861 = property on="Set from Input ch2" class="Bool"("DisabledEnum"=w3559) -> ()  [unwired: 2 in, 2 out]
        n1862 = property on="Set from Input ch4" class="Bool"("DisabledEnum"=w3559) -> ()  [unwired: 2 in, 2 out]
      }
      event "Copy to Input ch2": Value Change {
        w3594 = T12."Enabled" ("Disabled")
        n1863 = event-data() -> ()  [unwired: 1 in, 6 out]
        n1864 = call "Read AcquisitionB.vi"("error in (no error)"=w3627, "S4ACS_GUI in"=w3628) -> ("error out"=w3623:errorcluster, "Acquisition.lvclass"=w3626:refnum<class "Acquisition.lvclass">, "S4ACS_GUI out"=w3595:refnum<class "S4GUI.lvclass">)  [unwired: 7 in]
        n1865 = call-dynamic "Read Channel.vi"("error in (no error)"=w3623, "Acquisition in"=w3626) -> ("error out"=w3622:errorcluster, "Channel.lvclass"=w3625:refnum<class "Channel.lvclass">)  [unwired: 7 in, 1 out]
        n1866 = call-dynamic "Read Interface.vi"("error in (no error)"=w3622, "Channel in"=w3625) -> ("error out"=w3621:errorcluster, "Interface.lvclass"=w3624:refnum<class "Interface.lvclass">)  [unwired: 7 in, 1 out]
        n1867 = call-dynamic "Get CCD_Config.vi"("error in (no error)"=w3621, "Interface in"=w3624) -> ("error out"=w3618:errorcluster, "output cluster"=w3617:T31)  [unwired: 7 in, 1 out]
        n1868 = Unbundle By Name(w3617) -> ("INITIAL_LINE"=w3616:u16, "INITIAL_COLUMN"=w3615:u16, "FINAL_LINE"=w3614:u16, "FINAL_COLUMN"=w3613:u16, "VBIN"=w3612:u16, "HBIN"=w3611:u16, "PREAMP"=w3610:u8, "EM_GAIN"=w3609:u16, "READOUT_RATE"=w3608:u8, "SHUTTER_OPENING_TIME"=w3607:u16, "SHUTTER_CLOSING_TIME"=w3606:u16, "VERTICAL_SHIFT_SPEED"=w3605:u8, "READ_MODE"=w3604:u8, "VERTICAL_CLOCK_VOLTAGE"=w3603:u8, "AD_CHANNEL"=w3602:u32, "SHUTTER_MODE"=w3601:u8, "SHUTTER_TTL"=w3600:u8, "TRIGGER_MODE"=w3599:u8, "FRAME_TRANSFER"=w3598:bool, "ACQUISITION_MODE"=w3597:u8, "EM_MODE"=w3596:u8)
        n1869 = local read "Input Cluster"() -> (w3620:T8)
        n1870 = Bundle By Name(cluster=w3620, "Parameters.Image \nInitial Line"=w3616, "Parameters.Image\nInitial Column"=w3615, "Parameters.Image\nFinal Line"=w3614, "Parameters.Image\nFInal Column"=w3613, "Parameters.Vertical\nBinning"=w3612, "Parameters.Horizontal\nBinning"=w3611, "Parameters.Pre-amplification\nGain"=w3610, "Parameters.CCD\nEM Gain"=w3609, "Parameters.Readout\nRate"=w3608, "Parameters.Shutter\nOpenning Time"=w3607, "Parameters.Shutter\nClosing Time"=w3606, "Parameters.Vertical\nShift Speed"=w3605, "Parameters.Read\nMode"=w3604, "Parameters.Vertical\nClock Voltage"=w3603, "Parameters.A/D \nChannel"=w3602, "Parameters.Shutter\nMode"=w3601, "Parameters.Shutter\nTTL"=w3600, "Parameters.Trigger\nMode"=w3599, "Parameters.Frame\nTransfer"=w3598, "Parameters.Acquisition\nMode"=w3597, "Parameters.CCD \nEM Mode"=w3596) -> (w3619:T8)
        n1871 = local write "Input Cluster"(w3619) -> ()
        n1872 = property on="Set from Input ch1" class="Bool"("DisabledEnum"=w3594) -> ()  [unwired: 2 in, 2 out]
        n1873 = property on="Set from Input ch3" class="Bool"("DisabledEnum"=w3594) -> ()  [unwired: 2 in, 2 out]
        n1874 = property on="Set from Input ch2" class="Bool"("DisabledEnum"=w3594) -> ()  [unwired: 2 in, 2 out]
        n1875 = property on="Set from Input ch4" class="Bool"("DisabledEnum"=w3594) -> ()  [unwired: 2 in, 2 out]
      }
      event "Copy to Input ch3": Value Change {
        w3629 = T12."Enabled" ("Disabled")
        n1876 = event-data() -> ()  [unwired: 1 in, 6 out]
        n1877 = call-dynamic "Read AcquisitionC.vi"("error in (no error)"=w3662, "S4ACS_GUI in"=w3663) -> ("error out"=w3658:errorcluster, "Acquisition.lvclass"=w3661:refnum<class "Acquisition.lvclass">, "S4ACS_GUI out"=w3630:refnum<class "S4GUI.lvclass">)  [unwired: 7 in]
        n1878 = call-dynamic "Read Channel.vi"("error in (no error)"=w3658, "Acquisition in"=w3661) -> ("error out"=w3657:errorcluster, "Channel.lvclass"=w3660:refnum<class "Channel.lvclass">)  [unwired: 7 in, 1 out]
        n1879 = call-dynamic "Read Interface.vi"("error in (no error)"=w3657, "Channel in"=w3660) -> ("error out"=w3656:errorcluster, "Interface.lvclass"=w3659:refnum<class "Interface.lvclass">)  [unwired: 7 in, 1 out]
        n1880 = call-dynamic "Get CCD_Config.vi"("error in (no error)"=w3656, "Interface in"=w3659) -> ("error out"=w3653:errorcluster, "output cluster"=w3652:T31)  [unwired: 7 in, 1 out]
        n1881 = Unbundle By Name(w3652) -> ("INITIAL_LINE"=w3651:u16, "INITIAL_COLUMN"=w3650:u16, "FINAL_LINE"=w3649:u16, "FINAL_COLUMN"=w3648:u16, "VBIN"=w3647:u16, "HBIN"=w3646:u16, "PREAMP"=w3645:u8, "EM_GAIN"=w3644:u16, "READOUT_RATE"=w3643:u8, "SHUTTER_OPENING_TIME"=w3642:u16, "SHUTTER_CLOSING_TIME"=w3641:u16, "VERTICAL_SHIFT_SPEED"=w3640:u8, "READ_MODE"=w3639:u8, "VERTICAL_CLOCK_VOLTAGE"=w3638:u8, "AD_CHANNEL"=w3637:u32, "SHUTTER_MODE"=w3636:u8, "SHUTTER_TTL"=w3635:u8, "TRIGGER_MODE"=w3634:u8, "FRAME_TRANSFER"=w3633:bool, "ACQUISITION_MODE"=w3632:u8, "EM_MODE"=w3631:u8)
        n1882 = local read "Input Cluster"() -> (w3655:T8)
        n1883 = Bundle By Name(cluster=w3655, "Parameters.Image \nInitial Line"=w3651, "Parameters.Image\nInitial Column"=w3650, "Parameters.Image\nFinal Line"=w3649, "Parameters.Image\nFInal Column"=w3648, "Parameters.Vertical\nBinning"=w3647, "Parameters.Horizontal\nBinning"=w3646, "Parameters.Pre-amplification\nGain"=w3645, "Parameters.CCD\nEM Gain"=w3644, "Parameters.Readout\nRate"=w3643, "Parameters.Shutter\nOpenning Time"=w3642, "Parameters.Shutter\nClosing Time"=w3641, "Parameters.Vertical\nShift Speed"=w3640, "Parameters.Read\nMode"=w3639, "Parameters.Vertical\nClock Voltage"=w3638, "Parameters.A/D \nChannel"=w3637, "Parameters.Shutter\nMode"=w3636, "Parameters.Shutter\nTTL"=w3635, "Parameters.Trigger\nMode"=w3634, "Parameters.Frame\nTransfer"=w3633, "Parameters.Acquisition\nMode"=w3632, "Parameters.CCD \nEM Mode"=w3631) -> (w3654:T8)
        n1884 = local write "Input Cluster"(w3654) -> ()
        n1885 = property on="Set from Input ch1" class="Bool"("DisabledEnum"=w3629) -> ()  [unwired: 2 in, 2 out]
        n1886 = property on="Set from Input ch3" class="Bool"("DisabledEnum"=w3629) -> ()  [unwired: 2 in, 2 out]
        n1887 = property on="Set from Input ch2" class="Bool"("DisabledEnum"=w3629) -> ()  [unwired: 2 in, 2 out]
        n1888 = property on="Set from Input ch4" class="Bool"("DisabledEnum"=w3629) -> ()  [unwired: 2 in, 2 out]
      }
      event "Copy to Input ch4": Value Change {
        w3664 = T12."Enabled" ("Disabled")
        n1889 = event-data() -> ()  [unwired: 1 in, 6 out]
        n1890 = call-dynamic "Read AcquisitionD.vi"("error in (no error)"=w3697, "S4ACS_GUI in"=w3698) -> ("error out"=w3693:errorcluster, "Acquisition.lvclass"=w3696:refnum<class "Acquisition.lvclass">, "S4ACS_GUI out"=w3665:refnum<class "S4GUI.lvclass">)  [unwired: 7 in]
        n1891 = call-dynamic "Read Channel.vi"("error in (no error)"=w3693, "Acquisition in"=w3696) -> ("error out"=w3692:errorcluster, "Channel.lvclass"=w3695:refnum<class "Channel.lvclass">)  [unwired: 7 in, 1 out]
        n1892 = call-dynamic "Read Interface.vi"("error in (no error)"=w3692, "Channel in"=w3695) -> ("error out"=w3691:errorcluster, "Interface.lvclass"=w3694:refnum<class "Interface.lvclass">)  [unwired: 7 in, 1 out]
        n1893 = call-dynamic "Get CCD_Config.vi"("error in (no error)"=w3691, "Interface in"=w3694) -> ("error out"=w3688:errorcluster, "output cluster"=w3687:T31)  [unwired: 7 in, 1 out]
        n1894 = Unbundle By Name(w3687) -> ("INITIAL_LINE"=w3686:u16, "INITIAL_COLUMN"=w3685:u16, "FINAL_LINE"=w3684:u16, "FINAL_COLUMN"=w3683:u16, "VBIN"=w3682:u16, "HBIN"=w3681:u16, "PREAMP"=w3680:u8, "EM_GAIN"=w3679:u16, "READOUT_RATE"=w3678:u8, "SHUTTER_OPENING_TIME"=w3677:u16, "SHUTTER_CLOSING_TIME"=w3676:u16, "VERTICAL_SHIFT_SPEED"=w3675:u8, "READ_MODE"=w3674:u8, "VERTICAL_CLOCK_VOLTAGE"=w3673:u8, "AD_CHANNEL"=w3672:u32, "SHUTTER_MODE"=w3671:u8, "SHUTTER_TTL"=w3670:u8, "TRIGGER_MODE"=w3669:u8, "FRAME_TRANSFER"=w3668:bool, "ACQUISITION_MODE"=w3667:u8, "EM_MODE"=w3666:u8)
        n1895 = local read "Input Cluster"() -> (w3690:T8)
        n1896 = Bundle By Name(cluster=w3690, "Parameters.Image \nInitial Line"=w3686, "Parameters.Image\nInitial Column"=w3685, "Parameters.Image\nFinal Line"=w3684, "Parameters.Image\nFInal Column"=w3683, "Parameters.Vertical\nBinning"=w3682, "Parameters.Horizontal\nBinning"=w3681, "Parameters.Pre-amplification\nGain"=w3680, "Parameters.CCD\nEM Gain"=w3679, "Parameters.Readout\nRate"=w3678, "Parameters.Shutter\nOpenning Time"=w3677, "Parameters.Shutter\nClosing Time"=w3676, "Parameters.Vertical\nShift Speed"=w3675, "Parameters.Read\nMode"=w3674, "Parameters.Vertical\nClock Voltage"=w3673, "Parameters.A/D \nChannel"=w3672, "Parameters.Shutter\nMode"=w3671, "Parameters.Shutter\nTTL"=w3670, "Parameters.Trigger\nMode"=w3669, "Parameters.Frame\nTransfer"=w3668, "Parameters.Acquisition\nMode"=w3667, "Parameters.CCD \nEM Mode"=w3666) -> (w3689:T8)
        n1897 = local write "Input Cluster"(w3689) -> ()
        n1898 = property on="Set from Input ch1" class="Bool"("DisabledEnum"=w3664) -> ()  [unwired: 2 in, 2 out]
        n1899 = property on="Set from Input ch3" class="Bool"("DisabledEnum"=w3664) -> ()  [unwired: 2 in, 2 out]
        n1900 = property on="Set from Input ch2" class="Bool"("DisabledEnum"=w3664) -> ()  [unwired: 2 in, 2 out]
        n1901 = property on="Set from Input ch4" class="Bool"("DisabledEnum"=w3664) -> ()  [unwired: 2 in, 2 out]
      }
      event "Scrollbar": Value Change {
        (unwired) 765.0 ("BarOffset")
        (unwired) 1000.0 ("BarOffset")
        n1902 = event-data() -> ()  [unwired: 1 in, 6 out]
        n1903 = disable-structure shown="Disabled" {
          disable-tunnel: w3700 -> [w3712 _]
          frame Disabled {
            # "como alterar o valor de um parametro em \"Parameter Input\""
            n1904 = Unbundle By Name(w3712) -> ("Parameters"=w3714:T5)
            n1905 = Bundle By Name(cluster=w3714, "Readout\nRate"=u8 1 ("Readout\nRate")) -> (w3711:T5)
            n1906 = Bundle By Name(cluster=w3712, "Parameters"=w3711) -> (w3710:T8)
            n1907 = local write "Input Cluster"(w3710) -> ()
          }
          frame Enabled {
          }
        }
        n1908 = property on="Scrollbar" class="Scroll (strict)"() -> ("DocMax"=w3704:dbl)  [unwired: 2 in, 2 out]
        n1909 = Unbundle(w3702) -> ("Parameters"=w3707:refnum<vi>, "Current Configuration"=w3706:refnum<vi>)
        n1910 = Subtract(x=w3704, y="Scrollbar") -> (x-y=w3708:dbl)
        n1911 = Subtract(x=w3708, y=200.0 ("BarOffset")) -> (x-y=w3705:dbl)
        n1912 = property on="Property Node" class="Clust (strict)"(reference=w3707, "Top"=w3705) -> ()  [unwired: 1 in, 2 out]
        n1913 = property on="Property Node" class="Clust (strict)"(reference=w3706, "Top"=w3705) -> ()  [unwired: 1 in, 2 out]
      }
      event "Select Positions": Value Change {
        # "Garantir que, quando em POLARIMETRIA, pelo menos WP1 esteja selecionado."
        n1914 = event-data() -> ()  [unwired: 1 in, 6 out]
        n1915 = call "Read Instrument.lvclass.vi"("error in (no error)"=w3736, "S4ACS_GUI in"=w3735) -> ("error out"=w3745:errorcluster, "Instrument.lvclass"=w3744:refnum<class "Instrument.lvclass">, "S4ACS_GUI out"=w3738:refnum<class "S4GUI.lvclass">)  [unwired: 7 in]
        n1916 = call "Read WPROT.vi"("error in (no error)"=w3745, "Instrument in"=w3744) -> ("error out"=w3737:errorcluster, "Opt_Selector.lvclass"=w3741:refnum<class "Opt_Selector.lvclass">, "Instrument out"=w3739:refnum<class "Instrument.lvclass">)  [unwired: 7 in]
        n1917 = case shown="4" "Select Positions" {
          tunnel: w3737 -> [w3779 w3792 w3805 w3818 w3831 w3840]
          tunnel: [w3777 w3790 w3803 w3813 w3829 w3839] -> w3740
          tunnel: [w3774 w3788 w3801 w3815 w3827 w3840] -> w3733
          tunnel: w3741 -> [w3780 w3793 w3806 w3819 w3832 w3839]
          tunnel: [16 8 4 8 0 0] -> w3734
          tunnel: [0.0 ("Scale.Range:Minimum") 0.0 ("Scale.Range:Minimum") 0.0 ("Scale.Range:Minimum") 0.0 ("Scale.Range:Minimum") 0.0 ("Scale.Range:Minimum") 0.0 ("Scale.Range:Minimum")] -> w3732
          frame 0, Default {
            w3776 = u16 65535 ("sequencia")
            w3781 = TRUE ("P0")
            w3782 = TRUE ("P0")
            w3783 = TRUE ("P0")
            w3784 = TRUE ("P0")
            # "1111 1111 1111 1111 = 65.535"
            n1918 = local write "P0"(w3784) -> ()
            n1919 = local write "P1"(w3784) -> ()
            n1920 = local write "P2"(w3784) -> ()
            n1921 = local write "P3"(w3784) -> ()
            n1922 = local write "P4"(w3782) -> ()
            n1923 = local write "P5"(w3782) -> ()
            n1924 = local write "P6"(w3782) -> ()
            n1925 = local write "P7"(w3782) -> ()
            n1926 = call-dynamic "Write sequencia.vi"("error in (no error)"=w3779, "sequencia"=w3776, "Opt_Selector in"=w3780) -> ("error out"=w3775:errorcluster, "Opt_Selector out"=w3778:refnum<class "Opt_Selector.lvclass">)  [unwired: 7 in]
